vi "Error Dialog.vi"(8 "error in (no error)":errorcluster, 11 "RemoteControl in":refnum<class "RemoteControl.lvclass">) -> (0 "error out":errorcluster, 2 "States to Execute":string, 3 "RemoteControl out":refnum<class "RemoteControl.lvclass">)   [LabVIEW 2016, in "RemoteControl.lvclass"]
uses:
  RemoteControl.lvclass
  <userlib>/_OpenG.lib/error/error.llb/Filter Error Codes (Array)__ogtk.vi
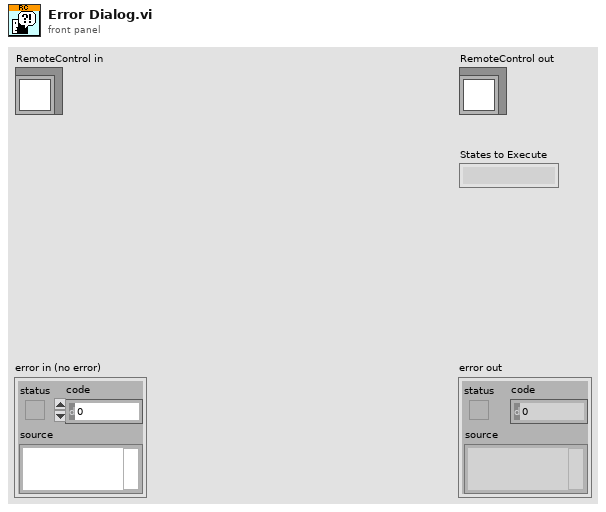
[diagram p1: front panel]
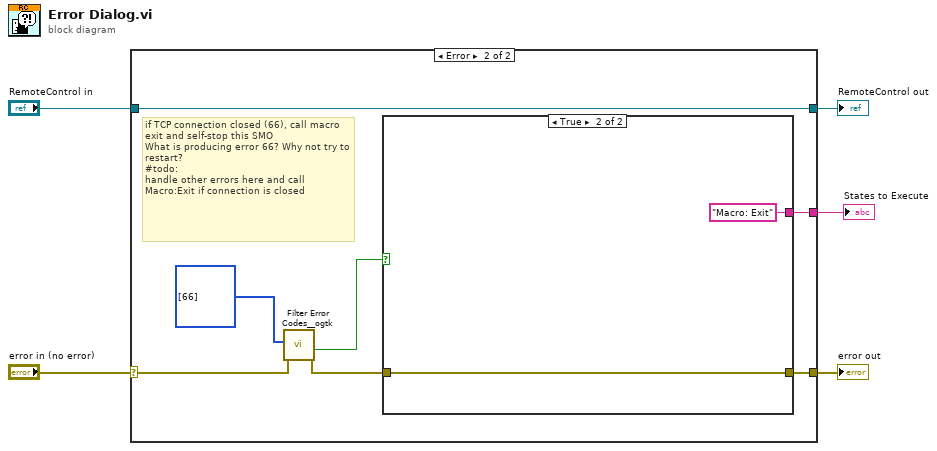
[diagram p0: block diagram]
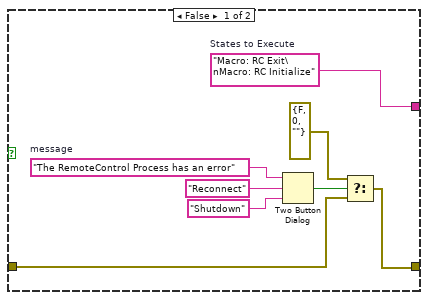
[diagram p3: hidden frame]
diagram:
  n1 = case shown="Error" "error in (no error)" {
    selector: "error in (no error)" -> [w6 w11]
    tunnel: [w6 w13] -> w4
    tunnel: [w7 w14] -> w2
    tunnel: "RemoteControl in" -> [w7 w14]
    tunnel: [_ w9] -> w1
    frame No Error {
      # "Wire the error cluster across even in the \"No Error\"\ncase so that warnings get propagated."
    }
    frame Error {
      # "if TCP connection closed (66), call macro exit and self-stop this SMO\nWhat is producing error 66? Why not try to restart?\n#todo:\nhandle other errors here and call\nMacro:Exit if connection is closed"
      n2 = call-poly <userlib>:"Filter Error Codes__ogtk.vi"("Error In"=w11, "Error Codes to Filter"=i32[] [66]) -> ("Error Out"=w10:errorcluster, "Error Filtered?"=w8:bool)  [unwired: 7 in, 1 out]
      n3 = case shown="True" w8 {
        tunnel: [w21 w24] -> w13
        tunnel: w10 -> [w16 w24]
        tunnel: [w15 "Macro: Exit" ("States to Execute")] -> w9
        frame False {
          w15 = "Macro: RC Exit\nMacro: RC Initialize"  # States to Execute
          w17 = "The RemoteControl Process has an error"  # message
          n4 = Two Button Dialog(message=w17, 1:"Shutdown" ("F button name (\"Cancel\")"), 2:"Reconnect" ("T button name (\"OK\")")) -> (T button?=w20:bool)
          n5 = Select(t=errorcluster {"status"=FALSE, "code"=0, "source"=""} ("error constant"), s=w20, f=w16) -> (s? t:f=w21:errorcluster)
        }
        frame True {
        }
      }
    }
  }
  "error out" <- w4
  "RemoteControl out" <- w2
  "States to Execute" <- w1
